vi "ConfigureTrig.vi"(8 "error in (no error)":errorcluster, 10 "TrigName":string, 11 "PXI_MultiTrig in":refnum<class "PXI_MultiTrig.lvclass">) -> (0 "error out":errorcluster, 3 "PXI_MultiTrig out":refnum<class "PXI_MultiTrig.lvclass">)   [LabVIEW 2018, in "SyncPlugins.lvlib" / "PXI_MultiTrig.lvclass"]
uses:
  PXI_MultiTrig.lvclass
  PXI_MultiTrig.lvclass/PXI_MultiTrig.ctl
  Accessors/Read RefClkSession.vi
  Accessors/Write Triggers.vi
  Accessors/Read TimingSession.vi
  Accessors/Read Triggers.vi
  <vilib>/Utility/error.llb/Error Cluster From Error Code.vi
  <vilib>/ErrorRing/Error Ring.xnode
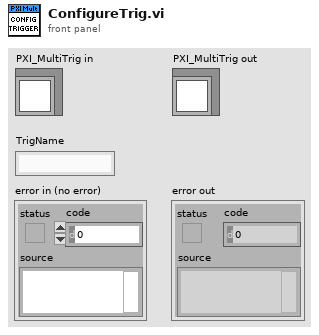
[diagram p1: front panel]
types:
  T1 = typedef "SyncPlugins.lvlib/PXI_MultiTrig.lvclass/clTrigger.ctl" = cluster{"Name":string, "DestTerm":string, "SrcTerm":string, "SyncClk":string, "Edge":i32, "Invert?":i32, "Initiated":bool, "Type":string, "TrigTime":bool}
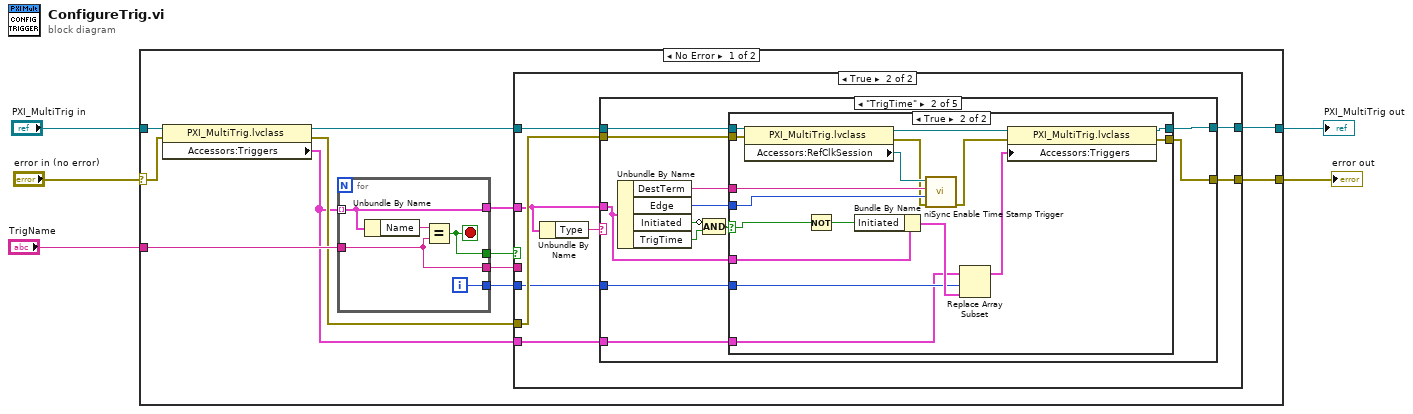
[diagram p0: block diagram]
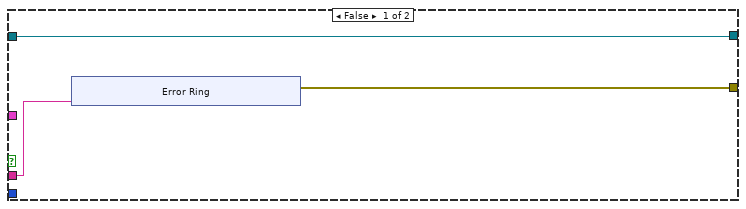
[diagram p2: hidden frame]
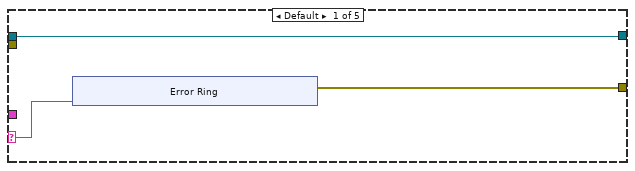
[diagram p3: hidden frame]
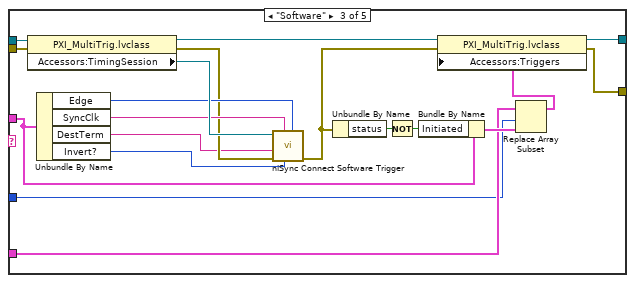
[diagram p5: hidden frame]
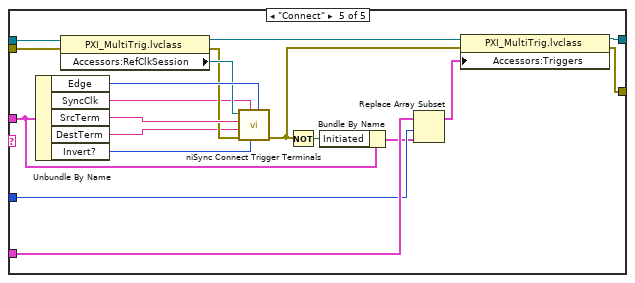
[diagram p7: hidden frame]
diagram:
  n1 = case shown="No Error" "error in (no error)" {
    selector: "error in (no error)" -> [w16 w123]
    tunnel: [w10 w123] -> w4
    tunnel: "PXI_MultiTrig in" -> [w17 w122]
    tunnel: [w8 w122] -> w2
    tunnel: "TrigName" -> [w15 _]
    frame No Error {
      n2 = property class="PXI_MultiTrig.lvclass"(reference=w17, error in=w16) -> (reference out=w14:refnum<class "PXI_MultiTrig.lvclass">, error out=w7:errorcluster, "Accessors:Triggers"=w6:T1[])
      n3 = for {
        tunnel: w6 -> [w120] mode=indexing
        tunnel: w15 -> [w118]
        tunnel: [w120] -> w9
        tunnel: [w119] -> w13
        tunnel: [w118] -> w12
        tunnel: [w117] -> w11
        i -> [w117]
        stop <- w119 stop-if-true
        n4 = Unbundle By Name(w120) -> ("Name"=w121:string)
        n5 = Equal?(x=w121, y=w118) -> (x = y?=w119:bool)
      }
      n6 = case shown="True" w13 {
        tunnel: w14 -> [w18 w35]
        tunnel: w12 -> [w20 _]
        tunnel: w11 -> [_ w28]
        tunnel: [w19 w32] -> w10
        tunnel: w9 -> [_ w30]
        tunnel: [w18 w34] -> w8
        tunnel: w7 -> [_ w33]
        tunnel: w6 -> [_ w29]
        frame False {
          n7 = xnode "Error Ring"("parameter 0"=w20) -> ("error out"=w19:errorcluster)
        }
        frame True {
          n8 = Unbundle By Name(w30) -> ("Type"=w31:string)
          n9 = case shown="\"TrigTime\"" w31 {
            selector: w31 -> [w37 _ _ _ _]
            tunnel: w35 -> [w38 w57 w95 w97 w115]
            tunnel: [w38 w50 w80 w97 w103] -> w34
            tunnel: w33 -> [_ w56 w93 w96 w114]
            tunnel: [w36 w49 w77 w96 w100] -> w32
            tunnel: w30 -> [_ w53 w83 _ w105]
            tunnel: w29 -> [_ w51 w82 _ w108]
            tunnel: w28 -> [_ w52 w81 _ w107]
            frame Default {
              n10 = xnode "Error Ring"("parameter 0"=w37) -> ("error out"=w36:errorcluster)
            }
            frame "TrigTime" {
              n11 = Unbundle By Name(w53) -> ("DestTerm"=w55:string, "Edge"=w54:i32, "Initiated"=w46:bool, "TrigTime"=w47:bool)
              n12 = Compound Arithmetic op=AND(invert w46, w47) -> (w48:bool)
              n13 = case shown="True" w48 {
                selector: w48 -> [_ w71]
                tunnel: w57 -> [w59 w76]
                tunnel: w56 -> [w58 w75]
                tunnel: w55 -> [_ w73]
                tunnel: w54 -> [_ w72]
                tunnel: w53 -> [_ w70]
                tunnel: w52 -> [_ w67]
                tunnel: w51 -> [_ w66]
                tunnel: [w59 w63] -> w50
                tunnel: [w58 w62] -> w49
                frame False {
                }
                frame True {
                  n14 = property class="PXI_MultiTrig.lvclass"(reference=w76, error in=w75) -> (reference out=w65:refnum<class "PXI_MultiTrig.lvclass">, error out=w61:errorcluster, "Accessors:RefClkSession"=w74:refnum<k15>)
                  n15 = Not(x=w71) -> (.not. x?=w69:bool)
                  n16 = Bundle By Name(cluster=w70, "Initiated"=w69) -> (w68:T1)
                  n17 = call <instrlib>:"niSync Enable Time Stamp Trigger.vi"("error in (no error)"=w61, "active edge"=w72, "terminal"=w73, "instrument handle"=w74) -> ("error out"=w60:errorcluster)  [unwired: 5 in, 1 out]
                  n18 = Replace Array Subset(array=w66, new element=w68, index=w67) -> (w64:T1[])
                  n19 = property class="PXI_MultiTrig.lvclass"(reference=w65, error in=w60, "Accessors:Triggers"=w64) -> (reference out=w63:refnum<class "PXI_MultiTrig.lvclass">, error out=w62:errorcluster)
                }
              }
            }
            frame "Software" {
              n20 = property class="PXI_MultiTrig.lvclass"(reference=w95, error in=w93) -> (reference out=w94:refnum<class "PXI_MultiTrig.lvclass">, error out=w89:errorcluster, "Accessors:TimingSession"=w92:refnum<k15>)
              n21 = Unbundle By Name(w83) -> ("Edge"=w90:i32, "SyncClk"=w91:string, "DestTerm"=w88:string, "Invert?"=w87:i32)
              n22 = call <instrlib>:"niSync Connect Software Trigger.vi"("update edge (Rising Edge)"=w90, "invert (Don't Invert Signal)"=w87, "synchronization clock"=w91, "error in (no error)"=w89, "destination terminal"=w88, "instrument handle"=w92) -> ("error out"=w78:errorcluster)  [unwired: 4 in, 1 out]
              n23 = Unbundle By Name(w78) -> ("status"=w86:bool)
              n24 = Not(x=w86) -> (.not. x?=w85:bool)
              n25 = Bundle By Name(cluster=w83, "Initiated"=w85) -> (w84:T1)
              n26 = Replace Array Subset(array=w82, new element=w84, index=w81) -> (w79:T1[])
              n27 = property class="PXI_MultiTrig.lvclass"(reference=w94, error in=w78, "Accessors:Triggers"=w79) -> (reference out=w80:refnum<class "PXI_MultiTrig.lvclass">, error out=w77:errorcluster)
            }
            frame "Timed" {
              # "Timed Triggers are configured by request.\nSee TimedTrigger.vi"
            }
            frame "Connect" {
              n28 = Unbundle By Name(w105) -> ("Edge"=w116:i32, "SyncClk"=w99:string, "SrcTerm"=w112:string, "DestTerm"=w98:string, "Invert?"=w110:i32)
              n29 = property class="PXI_MultiTrig.lvclass"(reference=w115, error in=w114) -> (reference out=w104:refnum<class "PXI_MultiTrig.lvclass">, error out=w111:errorcluster, "Accessors:RefClkSession"=w113:refnum<k15>)
              n30 = call <instrlib>:"niSync Connect Trigger Terminals.vi"("update edge (Rising Edge)"=w116, "invert (Don't Invert Signal)"=w110, "synchronization clock"=w99, "error in (no error)"=w111, "destination terminal"=w98, "source terminal"=w112, "instrument handle"=w113) -> ("error out"=w101:errorcluster)  [unwired: 3 in, 1 out]
              n31 = Not(x=w101) -> (.not. x?=w109:bool)
              n32 = Bundle By Name(cluster=w105, "Initiated"=w109) -> (w106:T1)
              n33 = Replace Array Subset(array=w108, new element=w106, index=w107) -> (w102:T1[])
              n34 = property class="PXI_MultiTrig.lvclass"(reference=w104, error in=w101, "Accessors:Triggers"=w102) -> (reference out=w103:refnum<class "PXI_MultiTrig.lvclass">, error out=w100:errorcluster)
            }
          }
        }
      }
    }
    frame Error {
    }
  }
  "error out" <- w4
  "PXI_MultiTrig out" <- w2
